vi "colored cells.vi"() -> ()   [LabVIEW 2024]
uses:
  Grid/SourceGrid.lvclass
  Views/Cell View/Cell View.lvclass
  System.Drawing.Color.ctl
  Cells/Cell/Cell.lvclass
  SourceGrid.lvlib
  D:/git/Sourcegrid-LabVIEW/dll/SourceGrid.dll
  dll/SourceGrid.dll
  D:/git/Sourcegrid-LabVIEW/source/Cells/Cell/Cell.lvclass
  D:/git/Sourcegrid-LabVIEW/source/ICloseable/ICloseable.lvclass
panel:
  in  "Grid Container":refnum<k24>(container)
  in  "stop":bool
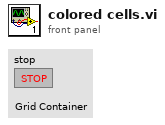
[diagram p1: front panel]
types:
  T1 = typedef "SourceGrid.lvlib/System.Drawing.Color.ctl" = enum16{"AliceBlue", "AntiqueWhite", "Aqua", "Aquamarine", "Azure", "Beige", "Bisque", "Black", "BlanchedAlmond", "Blue", "BlueViolet", "Brown", "BurlyWood", "CadetBlue", "Chartreuse", "Chocolate", "Coral", "CornflowerBlue", "Cornsilk", "Crimson", "Cyan", "DarkBlue", "DarkCyan", "DarkGoldenrod", "DarkGray", "DarkGreen", "DarkKhaki", "DarkMagenta", "DarkOliveGreen", "DarkOrange", "DarkOrchid", "DarkRed", "DarkSalmon", "DarkSeaGreen", "DarkSlateBlue", "DarkSlateGray", "DarkTurquoise", "DarkViolet", "DeepPink", "DeepSkyBlue", "DimGray", "DodgerBlue", "Firebrick", "FloralWhite", "ForestGreen", "Fuchsia", "Gainsboro", "GhostWhite", "Gold", "Goldenrod", "Gray", "Green", "GreenYellow", "Honeydew", "HotPink", "IndianRed", "Indigo", "Ivory", "Khaki", "Lavender", "LavenderBlush", "LawnGreen", "LemonChiffon", "LightBlue", "LightCoral", "LightCyan", "LightGoldenrodYellow", "LightGray", "LightGreen", "LightPink", "LightSalmon", "LightSeaGreen", "LightSkyBlue", "LightSlateGray", "LightSteelBlue", "LightYellow", "Lime", "LimeGreen", "Linen", "Magenta", "Maroon", "MediumAquamarine", "MediumBlue", "MediumOrchid", "MediumPurple", "MediumSeaGreen", "MediumSlateBlue", "MediumSpringGreen", "MediumTurquoise", "MediumVioletRed", "MidnightBlue", "MintCream", "MistyRose", "Moccasin", "NavajoWhite", "Navy", "OldLace", "Olive", "OliveDrab", "Orange", "OrangeRed", "Orchid", "PaleGoldenrod", "PaleGreen", "PaleTurquoise", "PaleVioletRed", "PapayaWhip", "PeachPuff", "Peru", "Pink", "Plum", "PowderBlue", "Purple", "Red", "RosyBrown", "RoyalBlue", "SaddleBrown", "Salmon", "SandyBrown", "SeaGreen", "SeaShell", "Sienna", "Silver", "SkyBlue", "SlateBlue", "SlateGray", "Snow", "SpringGreen", "SteelBlue", "Tan", "Teal", "Thistle", "Tomato", "Transparent", "Turquoise", "Violet", "Wheat", "White", "WhiteSmoke", "Yellow"}
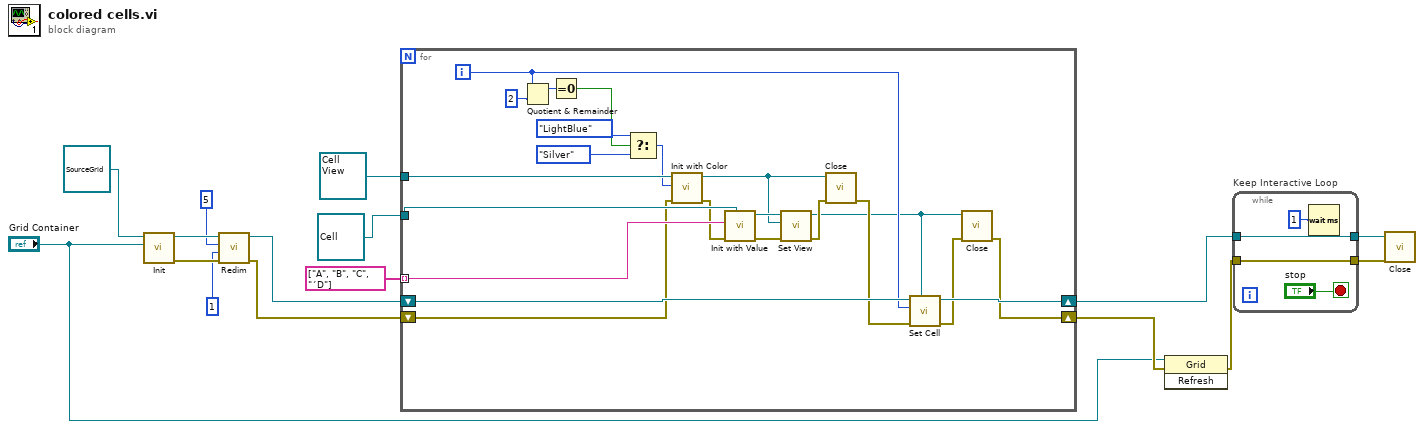
[diagram p0: block diagram]
diagram:
  n1 = call-dynamic "Init.vi"("Sourcegrid Container"="Grid Container", "Grid in"=refnum<class "SourceGrid.lvclass"> refnum) -> ("error out"=w13:errorcluster, "Grid out"=w11:refnum<class "SourceGrid.lvclass">)  [unwired: 8 in]
  n2 = call "Redim.vi"("error in"=w13, "Columns"=1, "Rows"=5, "Sourcegrid in"=w11) -> ("error out"=w8:errorcluster, "Sourcegrid out"=w7:refnum<class "SourceGrid.lvclass">)  [unwired: 6 in]
  n3 = for {
    shift-right: [w25] -> w12
    shift-left: w7 -> [w37]
    shift-right: [w17] -> w6
    shift-left: w8 -> [w24]
    tunnel: refnum<class "Cell View.lvclass"> refnum ("Cell View in") -> [w36]
    tunnel: refnum<class "Cell.lvclass"> refnum ("Cell in") -> [w35]
    tunnel: string[] ["A", "B", "C", "´D"] -> [w34] mode=indexing
    i -> [w33]
    n4 = Quotient & Remainder(x=w33, y=2) -> (x-y*floor(x/y)=w31:i32)  [unwired: 1 out]
    n5 = Equal To 0?(x=w31) -> (x = 0?=w30:bool)
    n6 = Select(t=System.Drawing.Color."LightBlue" ("Color"), s=w30, f=System.Drawing.Color."Silver" ("Color")) -> (s? t:f=w29:T1)
    n7 = call-dynamic "Init with Color.vi"("error in"=w24, "Color"=w29, "Cell View in"=w36) -> ("error out"=w23:errorcluster, "Cell View out"=w22:refnum<class "Cell View.lvclass">)  [unwired: 7 in]
    n8 = call-dynamic "Init with Value.vi"(7:w35, "error in"=w23, "Value"=w34) -> ("error out"=w38:errorcluster, "Cell out"=w26:refnum<class "Cell.lvclass">)  [unwired: 7 in]
    n9 = call-dynamic "Set View.vi"("error in"=w38, "CellView"=w22, "Cell in"=w26) -> ("error out"=w21:errorcluster, "Cell out"=w18:refnum<class "Cell.lvclass">)  [unwired: 7 in]
    n10 = call-dynamic "Close.vi"("error in"=w21, "Cell View in"=w22) -> ("error out"=w20:errorcluster)  [unwired: 8 in, 1 out]
    n11 = call "Set Cell.vi"("Cell"=w18, "error in"=w20, "Row"=w33, "Sourcegrid in"=w37) -> ("error out"=w19:errorcluster, "Sourcegrid out"=w25:refnum<class "SourceGrid.lvclass">)  [unwired: 6 in]
    n12 = call-dynamic "Close.vi"("error in"=w19, "Cell in"=w18) -> ("error out"=w17:errorcluster)  [unwired: 8 in, 1 out]
  }
  n13 = invoke class="Grid" method="Refresh"(reference="Grid Container", error in=w6) -> (error out=w5:errorcluster)  [unwired: 1 in, 2 out]
  n14 = while "Keep Interactive Loop" {
    tunnel: w12 -> [w42]
    tunnel: [w42] -> w16
    tunnel: w5 -> [w41]
    tunnel: [w41] -> w15
    stop <- "stop" stop-if-true
    n15 = Wait (ms)(milliseconds to wait=u32 1) -> ()  [unwired: 1 out]
  }
  n16 = call-dynamic "Close.vi"("error in"=w15, "Sourcegrid in"=w16) -> ()  [unwired: 8 in, 2 out]
